vi "Write FPSZ.vi"(3 "FP":refnum<class "DecFrame_FP.lvclass">, 4 "FPSZ":refnum<class "GObject_FPSZ.lvclass">) -> (5 "FP Out":refnum<class "DecFrame_FP.lvclass">)   [LabVIEW 2025, in "DecFrame_FP.lvclass"]
uses:
  DecFrame_FP/DecFrame_FP.lvclass
  GObject_FPSZ/GObject_FPSZ.lvclass
  DecFrame_FP/DecFrame_FP.lvclass/DecFrame_FP.ctl
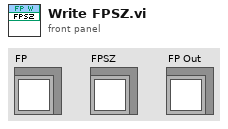
[diagram p1: front panel]
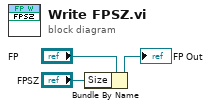
[diagram p0: block diagram]
diagram:
  n1 = Bundle By Name(cluster="FP", "Size"="FPSZ") -> (→"FP Out":refnum<class "DecFrame_FP.lvclass">)
